vi "Send stimulus trigger setup.vi"(8 "error in (no error)":errorcluster, 11 "FPGA ref in":T1) -> (0 "error out":errorcluster, 3 "FPGA ref out":T1)   [LabVIEW 2020]
uses:
  RIG-SPECIFIC FILES/FPGA Refs/FPGA Ref.ctl
  typedefs/Stimulus trigger delays cluster.ctl
  <vilib>/Utility/error.llb/Error Cluster From Error Code.vi
  <vilib>/rvi/errors/niLvFpgaAdjustHostInterfaceError.vi
  <vilib>/rvi/interface/nirviReadWriteControl/nirviReadWriteControl.xnode
  NiFpgaLv.dll
  <vilib>/rvi/interface/Simulation/niFpgaSimulationCallBeginRW.vi
panel:
  out "Enable stimulus?":bool
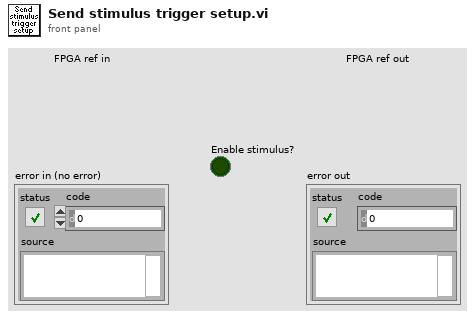
[diagram p1: front panel]
types:
  T1 = typedef "FPGA Ref.ctl" = refnum<k20>
  T2 = typedef "Stimulus trigger delays cluster.ctl" = cluster{"Trigger period in live protocols (80MHz Cycles)":u32, "Pulse width in live protocols (80MHz Cycles)":u32, "Enable stimulus in live protocols":bool, "Trigger delay in funct. protocols (80MHz Cycles)":u32, "Pulse width in funct. protocols (80MHz Cycles)":u32, "Enable stimulus in funct. protocols":bool}
  T3 = typedef "AOL_Globals.ctl" = cluster{"Imaging Protocol":T4, "Number of POI":u16, "Number of Miniscans":u16, "Number of Trials":u16, "Number of Cycles ":u64, "# Averaged Frames":u16, "Laser power (%)":u8, "Pockels (V)":dbl, "Acquisition Length (sec)":dbl, "Fill time (us)":dbl, "POI Dwell time (us)":dbl, "Miniscan Dwell time per pixel (us)":dbl, "PMT 1":dbl, "PMT 2":dbl, "Back Apperture (mA)":dbl, "Frame Size":T5, "Center Frequency":dbl, "Field of View (um)":dbl, "Field of View (norm)":dbl, "DwellTime (us)":dbl, "Ref Dwell Time (us)":dbl, "Wavelength (nm)":dbl, "Zoom":dbl, "AOL Z":dbl, "AOL Mode":T6, "GridXY":dbl, "GridZ":dbl, "TriggerPeriod (sec)":dbl, "Number of Pixels in Miniscan":u16, "Experiment folder path":path, "X centre":dbl, "Y centre":dbl, "Angle (degrees)":dbl, "Angle Xs (degrees)":dbl, "Angle Ys (degrees)":dbl, "Plane Mode":T7, "Threshold":u16[], "Regenerate Chirps":bool, "Rectangle ROI length (pixels)":u16, "Rectangle ROI height (pixels)":u16, "AOD fill":u16, "StartupDelay":i32, "Samples Wait after Trigger":u16, "Slip Cycle":u32, "Add Cycle":bool, "Functional Mode":T8, "Z Start":dbl, "Z Stop":dbl, "# Planes":i32, "Total Pixels":i32, "Variable Miniscan Pixels":u16[], "Use Variable Length":bool, "Use Variable Resolution":bool, "Laser power (%) at Z Start":u8, "Laser power (%) at Z Stop":u8, "Ref Z Step":i8}
  T4 = typedef "Imaging Protocols enum.ctl" = enum16{"AOL Z-Stack", "Motor Z Stack", "Parameter Sweep", "Functional Acquisition", "Single Plane Acquisition", "Volume Acquisition", "Live Imaging", "Live Plane Imaging", "Live Volume Imaging"}
  T5 = typedef "Frame Size.ctl" = u16
  T6 = typedef "AOL modes.ctl" = enum16{"Raster", "Structural", "Pointing", "Mini Scan", "Alignment"}
  T7 = typedef "Plane Mode.ctl" = u16
  T8 = typedef "Functional Mode.ctl" = enum16{"Point", "Line", "Patch", "Plane", "Volume"}
  T9 = enum16{"AOL Z-Stack", "Motor Z Stack", "Functional Acquisition", "Single Plane Acquisition", "Volume Acquisition", "Live Imaging", "Live Plane Imaging", "Live Volume Imaging"}
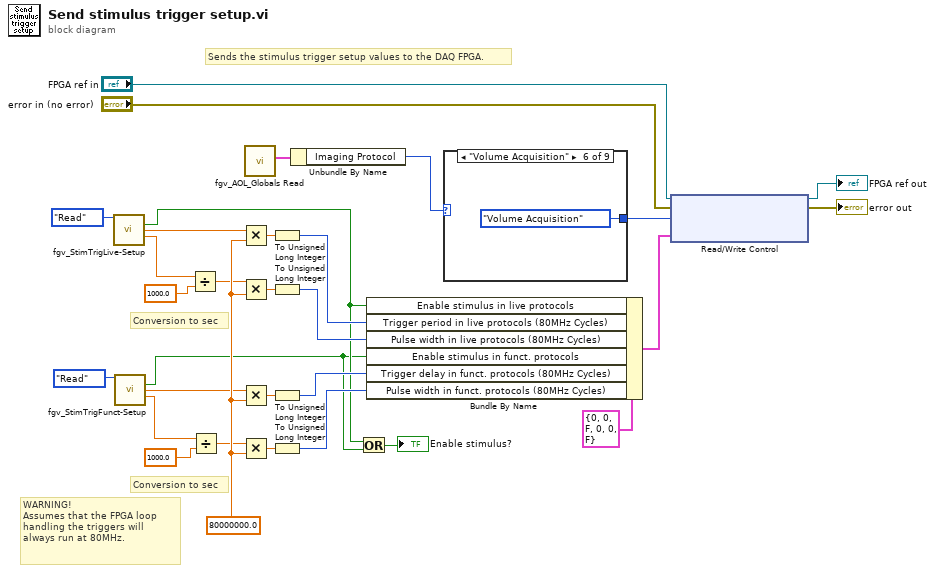
[diagram p0: block diagram]
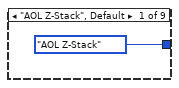
[diagram p2: hidden frame]
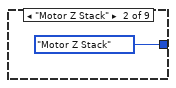
[diagram p3: hidden frame]
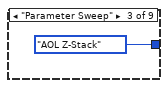
[diagram p4: hidden frame]
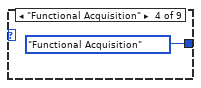
[diagram p5: hidden frame]
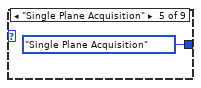
[diagram p6: hidden frame]
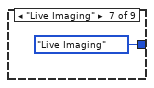
[diagram p7: hidden frame]
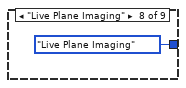
[diagram p8: hidden frame]
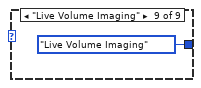
[diagram p9: hidden frame]
diagram:
  w17 = 80000000.0 ("Delay in live protocols (80MHz Cycles)")
  # "Conversion to sec"
  # "Conversion to sec"
  # "WARNING!\nAssumes that the FPGA loop handling the triggers will always run at 80MHz."
  # "Sends the stimulus trigger setup values to the DAQ FPGA."
  n1 = call "fgv_StimTrigLive-Setup.vi"("Function"=enum16{"Intialize", "Write", "Read", "Clear"}."Read") -> ("Live stim.trig.enable"=w12:bool, "Live stim.trig.period (sec)"=w7:dbl, "Live stim.trig.width (ms)"=w8:dbl)  [unwired: 11 in, 1 out]
  n2 = call "fgv_StimTrigFunct-Setup.vi"("Function"=enum16{"Intialize", "Write", "Read", "Clear"}."Read") -> ("Funct stim.trig.enable"=w11:bool, "Funct stim.trig.delay (sec)"=w5:dbl, "Funct stim.trig.width (ms)"=w9:dbl)  [unwired: 11 in, 1 out]
  n3 = Divide(x=w8, y=1000.0) -> (x/y=w6:dbl)
  n4 = Divide(x=w9, y=1000.0) -> (x/y=w4:dbl)
  n5 = Multiply(x=w7, y=w17) -> (x*y=w25:dbl)
  n6 = Multiply(x=w6, y=w17) -> (x*y=w27:dbl)
  n7 = Multiply(x=w5, y=w17) -> (x*y=w23:dbl)
  n8 = Multiply(x=w4, y=w17) -> (x*y=w18:dbl)
  n9 = call "fgv_AOL_Globals Read.vi"() -> ("AOL_Globals"=w22:T3)  [unwired: 9 in, 2 out]
  n10 = To Unsigned Long Integer(number=w25) -> (unsigned 32bit integer=w16:u32)
  n11 = To Unsigned Long Integer(number=w27) -> (unsigned 32bit integer=w14:u32)
  n12 = To Unsigned Long Integer(number=w23) -> (unsigned 32bit integer=w15:u32)
  n13 = To Unsigned Long Integer(number=w18) -> (unsigned 32bit integer=w13:u32)
  n14 = Unbundle By Name(w22) -> ("Imaging Protocol"=w2:T4)
  n15 = Or(x=w12, y=w11) -> (x .or. y?=→"Enable stimulus?":bool)
  n16 = Bundle By Name(cluster=T2 {"Trigger period in live protocols (80MHz Cycles)"=0, "Pulse width in live protocols (80MHz Cycles)"=0, "Enable stimulus in live protocols"=FALSE, "Trigger delay in funct. protocols (80MHz Cycles)"=0, "Pulse width in funct. protocols (80MHz Cycles)"=0, "Enable stimulus in funct. protocols"=FALSE} ("Trigger delays"), "Enable stimulus in live protocols"=w12, "Trigger period in live protocols (80MHz Cycles)"=w16, "Pulse width in live protocols (80MHz Cycles)"=w14, "Enable stimulus in funct. protocols"=w11, "Trigger delay in funct. protocols (80MHz Cycles)"=w15, "Pulse width in funct. protocols (80MHz Cycles)"=w13) -> (w26:T2)
  n17 = case shown="\"Volume Acquisition\"" w2 {
    tunnel: [T9."AOL Z-Stack" ("Imaging Protocol") T9."Motor Z Stack" ("Imaging Protocol") T9."AOL Z-Stack" ("Imaging Protocol") T9."Functional Acquisition" ("Imaging Protocol") T9."Single Plane Acquisition" ("Imaging Protocol") T9."Volume Acquisition" ("Imaging Protocol") T9."Live Imaging" ("Imaging Protocol") T9."Live Plane Imaging" ("Imaging Protocol") T9."Live Volume Imaging" ("Imaging Protocol")] -> w1
    frame "AOL Z-Stack", Default {
    }
    frame "Motor Z Stack" {
    }
    frame "Parameter Sweep" {
    }
    frame "Functional Acquisition" {
    }
    frame "Single Plane Acquisition" {
    }
    frame "Volume Acquisition" {
    }
    frame "Live Imaging" {
    }
    frame "Live Plane Imaging" {
    }
    frame "Live Volume Imaging" {
    }
  }
  n18 = xnode ("Read/Write Control")("FPGA VI Reference In"="FPGA ref in", "error in"="error in (no error)", "Imaging Protocol"=w1, "Stimulus Trigger Setup"=w26) -> ("FPGA VI Reference Out"=→"FPGA ref out":T1, "error out"=→"error out":errorcluster)
